vi "Configure Marker Type.vi"   [LabVIEW 2018, in "Agilent MXA Series.lvlib"]
doc: "Configures the marker type on the spectrum analyzer."
uses:
  Agilent MXA Series.lvlib
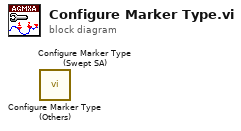
[diagram p0: block diagram]
diagram:
  n1 = call "Configure Marker Type (Others).vi"() -> ()  [unwired: 14 in, 2 out]
  n2 = call "Configure Marker Type (Swept SA).vi"() -> ()  [unwired: 14 in, 2 out]
